vi "Read class timings.vi"(8 "error in (no error)":errorcluster, 11 "Simulated Camera in":refnum<class "Sim_CCD.lvclass">) -> (0 "error out":errorcluster, 2 "class timings":T2, 3 "Simulated Camera out":refnum<class "Sim_CCD.lvclass">)   [LabVIEW 2018, in "Sim_CCD.lvclass"]
uses:
  Sim_CCD.lvclass
  <vilib>/Utility/miscctls.llb/LVDateTimeRec.ctl
  Sim_CCD.lvclass/Sim_CCD.ctl
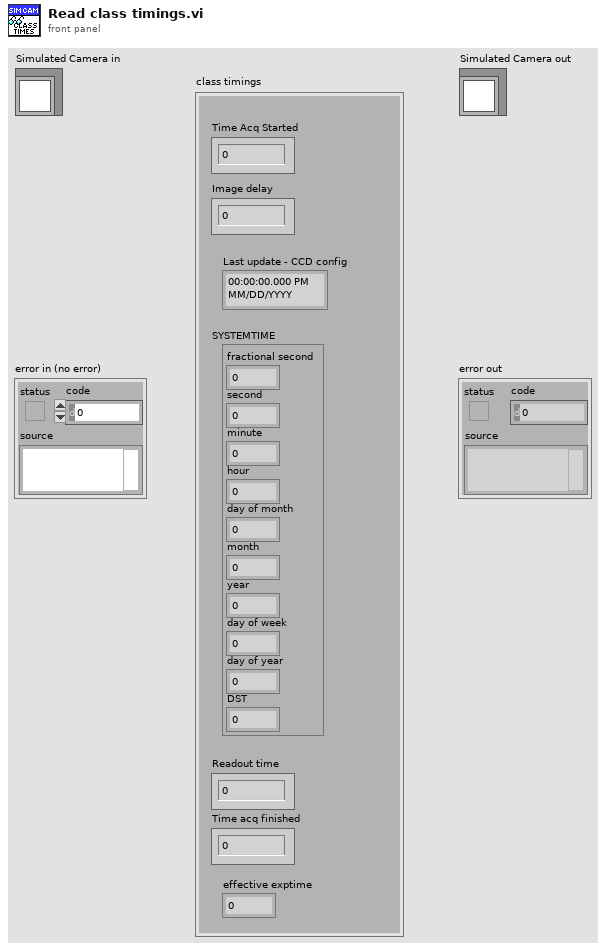
[diagram p1: front panel]
types:
  T1 = typedef "LVDateTimeRec.ctl" = cluster{"fractional second":dbl, "second":i32, "minute":i32, "hour":i32, "day of month":i32, "month":i32, "year":i32, "day of week":i32, "day of year":i32, "DST":i32}
  T2 = cluster{"Time Acq Started":u32, "Image delay":u64, "Last update - CCD config":timestamp, "SYSTEMTIME":T1, "Readout time":dbl, "Time acq finished":u32, "effective exptime":dbl}
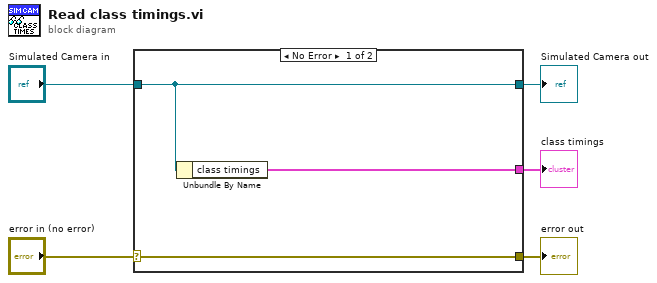
[diagram p0: block diagram]
diagram:
  n1 = case shown="No Error" "error in (no error)" {
    selector: "error in (no error)" -> [w8 w9]
    tunnel: [w8 w9] -> w4
    tunnel: [w7 w10] -> w2
    tunnel: "Simulated Camera in" -> [w7 w10]
    tunnel: [w6 _] -> w1
    frame No Error {
      n2 = Unbundle By Name(w7) -> ("class timings"=w6:T2)
    }
    frame Error {
    }
  }
  "error out" <- w4
  "Simulated Camera out" <- w2
  "class timings" <- w1
